vi "Arquivo de Configuração.vi"(0 "Caminho do arquivo":path, 1 "Modo":T2, 2 "Configurações":T1={"Simulações"={"Nível Qualidade"="avi", "Turno"="avi"}, "Captura de Imagens"={"Pasta com imagens"=path "", "Mostrar imagens capturadas"=FALSE}, "Caminhos"={"Arquivo de configuração"=path ""}}, 3 "error in (no error)":errorcluster) -> (9 "Configurações 2":T1={"Simulações"={"Nível Qualidade"="avi", "Turno"="avi"}, "Captura de Imagens"={"Pasta com imagens"=path "", "Mostrar imagens capturadas"=FALSE}, "Caminhos"={"Arquivo de configuração"=path ""}}, 10 "error out":errorcluster)   [LabVIEW 2020, in "Configurações.lvlib"]
uses:
  <vilib>/Utility/config.llb/Read Key (I32).vi
  <vilib>/Utility/config.llb/Write Key (I32).vi
  <vilib>/Utility/config.llb/Read Key (Path).vi
  <vilib>/Utility/config.llb/Write Key (Path).vi
  <vilib>/Utility/config.llb/Read Key (Boolean).vi
  <vilib>/Utility/config.llb/Write Key (Boolean).vi
  <vilib>/Utility/config.llb/Read Key (String).vi
  <vilib>/Utility/config.llb/Write Key (String).vi
  <vilib>/Utility/config.llb/NI_LVConfig.lvlib
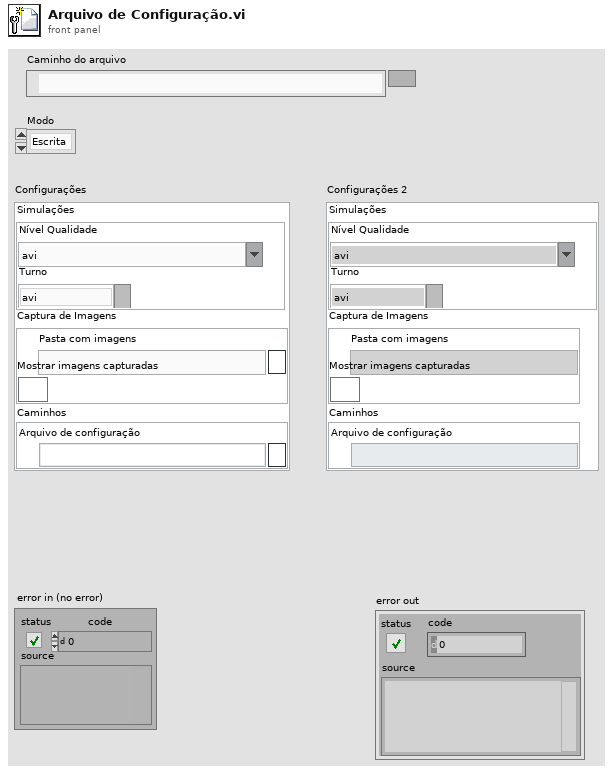
[diagram p1: front panel]
types:
  T1 = typedef "Configurações.lvlib/Configurações padrões.ctl" = cluster{"Simulações":cluster{"Nível Qualidade":string, "Turno":string}, "Captura de Imagens":cluster{"Pasta com imagens":path, "Mostrar imagens capturadas":bool}, "Caminhos":cluster{"Arquivo de configuração":path}}
  T2 = typedef "Ações de configuração 2.ctl" = enum16{"Escrita", "Leitura"}
  T3 = typedef "NI_LVConfig.lvlib/Config Data RefNum.ctl" = refnum<k1>
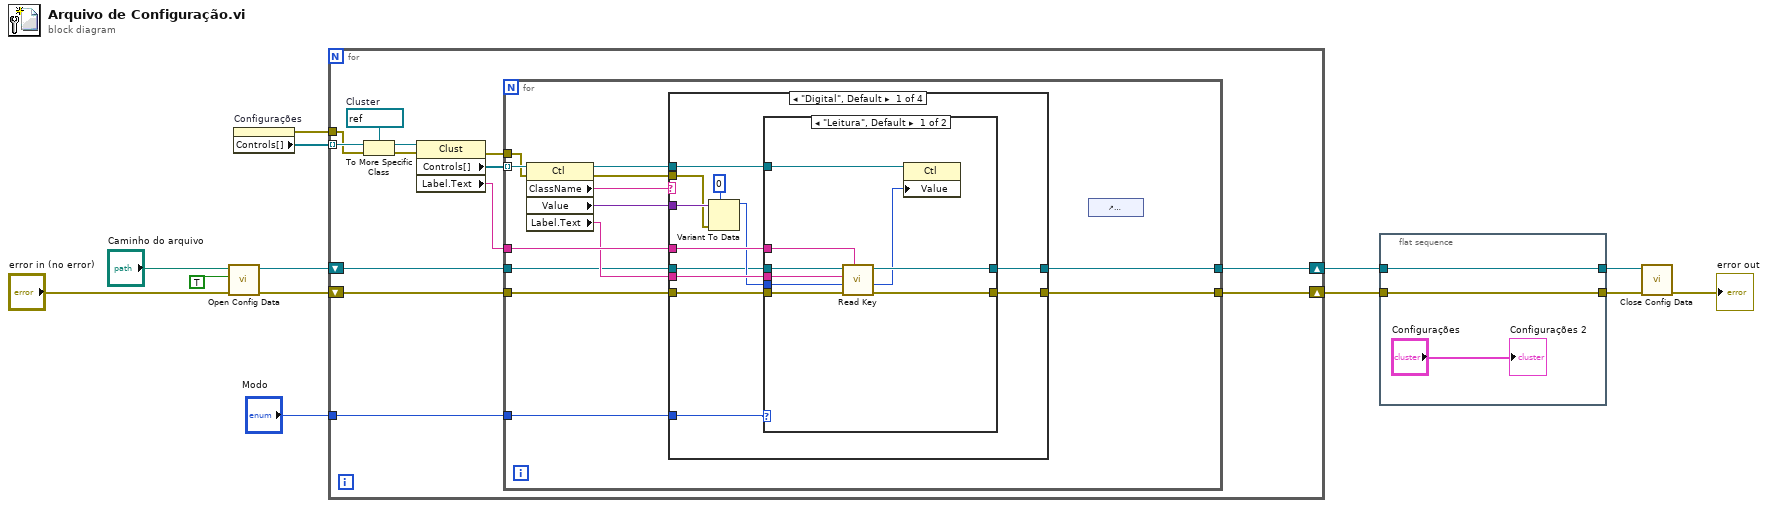
[diagram p0: block diagram]
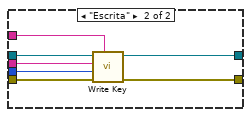
[diagram p2: hidden frame]
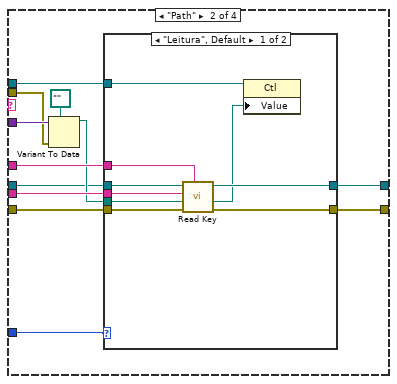
[diagram p3: hidden frame]
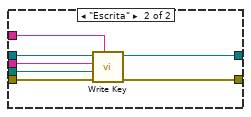
[diagram p4: hidden frame]
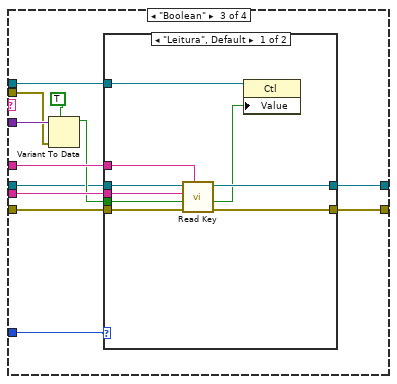
[diagram p5: hidden frame]
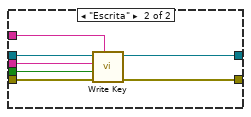
[diagram p6: hidden frame]
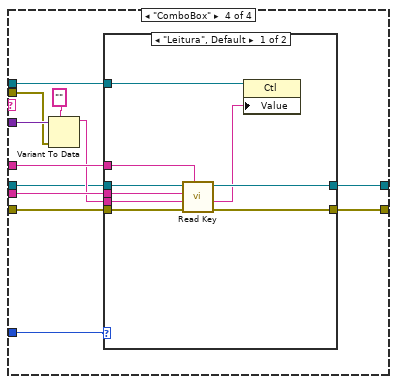
[diagram p7: hidden frame]
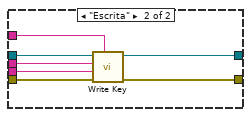
[diagram p8: hidden frame]
diagram:
  n1 = call <vilib>:"Open Config Data.vi"("error in (no error)"="error in (no error)", "create file if necessary (T)"=TRUE, "configuration file path"="Caminho do arquivo") -> ("error out"=w11:errorcluster, "refnum"=w12:T3)  [unwired: 6 in, 1 out]
  n2 = property on="Configurações" class="Clust (strict)"() -> (error out=w5:errorcluster, "Controls[]"=w9:refnum<vi>[])  [unwired: 2 in, 1 out]
  n3 = for {
    shift-right: [w18] -> w3
    shift-left: w12 -> [w19]
    shift-right: [w16] -> w1
    shift-left: w11 -> [w17]
    tunnel: w9 -> [w25] mode=indexing
    tunnel: "Modo" -> [w15]
    tunnel: w5 -> [w14]
    w26 = refnum<vi> refnum  # Cluster
    n4 = To More Specific Class(target class=w26, reference=w25, error in=w14) -> (specific class reference=w24:refnum<vi>, error out=w23:errorcluster)
    n5 = property class="Clust"(reference=w24, error in=w23) -> (error out=w21:errorcluster, "Controls[]"=w22:refnum<vi>[], "Label.Text"=w20:string)  [unwired: 1 out]
    n6 = for {
      tunnel: w22 -> [w39] mode=indexing
      tunnel: w21 -> [w36]
      tunnel: w20 -> [w34]
      tunnel: w19 -> [w32]
      tunnel: [w31] -> w18
      tunnel: w17 -> [w30]
      tunnel: [w29] -> w16
      tunnel: w15 -> [w28]
      n7 = property class="Ctl"(reference=w39, error in=w36) -> (reference out=w27:refnum<vi>, error out=w35:errorcluster, "ClassName"=w38:string, "Value"=w37:variant, "Label.Text"=w33:string)
      n8 = case shown="\"Digital\", Default" w38 {
        tunnel: w37 -> [w51 w79 w107 w135]
        tunnel: w35 -> [w50 w78 w106 w134]
        tunnel: w34 -> [w49 w77 w105 w133]
        tunnel: w33 -> [w48 w76 w104 w132]
        tunnel: w32 -> [w46 w74 w102 w130]
        tunnel: [w45 w73 w101 w129] -> w31
        tunnel: w30 -> [w44 w72 w100 w128]
        tunnel: [w43 w71 w99 w127] -> w29
        tunnel: w28 -> [w41 w70 w98 w126]
        tunnel: w27 -> [w40 w69 w97 w125]
        frame "Digital", Default {
          n9 = Variant To Data(error in=w50, type=0, Variant=w51) -> (data=w47:i32)  [unwired: 1 out]
          n10 = case shown="\"Leitura\", Default" w41 {
            tunnel: w49 -> [w53 w67]
            tunnel: w48 -> [w52 w66]
            tunnel: w47 -> [w56 w65]
            tunnel: w46 -> [w60 w64]
            tunnel: [w59 w63] -> w45
            tunnel: w44 -> [w58 w62]
            tunnel: [w57 w61] -> w43
            tunnel: w40 -> [w55 _]
            frame "Leitura", Default {
              n11 = call-poly <vilib>:"Read Key.vi"("section"=w53, "error in (no error)"=w58, "default value"=w56, "key"=w52, "refnum"=w60) -> ("error out"=w57:errorcluster, "value"=w54:i32, "refnum out"=w59:T3)  [unwired: 3 in, 1 out]
              n12 = property class="Ctl"(reference=w55, "Value"=w54) -> ()  [unwired: 1 in, 2 out]
            }
            frame "Escrita" {
              n13 = call-poly <vilib>:"Write Key.vi"("section"=w67, "error in (no error)"=w62, "value"=w65, "key"=w66, "refnum"=w64) -> ("error out"=w61:errorcluster, "refnum out"=w63:T3)  [unwired: 4 in, 1 out]
            }
          }
        }
        frame "Path" {
          n14 = Variant To Data(error in=w78, type=path "", Variant=w79) -> (data=w75:path)  [unwired: 1 out]
          n15 = case shown="\"Leitura\", Default" w70 {
            tunnel: w77 -> [w81 w95]
            tunnel: w76 -> [w80 w94]
            tunnel: w75 -> [w84 w93]
            tunnel: w74 -> [w88 w92]
            tunnel: [w87 w91] -> w73
            tunnel: w72 -> [w86 w90]
            tunnel: [w85 w89] -> w71
            tunnel: w69 -> [w83 _]
            frame "Leitura", Default {
              n16 = call-poly <vilib>:"Read Key.vi"("section"=w81, "error in (no error)"=w86, "default value"=w84, "key"=w80, "refnum"=w88) -> ("error out"=w85:errorcluster, "value"=w82:path, "refnum out"=w87:T3)  [unwired: 3 in, 1 out]
              n17 = property class="Ctl"(reference=w83, "Value"=w82) -> ()  [unwired: 1 in, 2 out]
            }
            frame "Escrita" {
              n18 = call-poly <vilib>:"Write Key.vi"("section"=w95, "error in (no error)"=w90, "value"=w93, "key"=w94, "refnum"=w92) -> ("error out"=w89:errorcluster, "refnum out"=w91:T3)  [unwired: 4 in, 1 out]
            }
          }
        }
        frame "Boolean" {
          n19 = Variant To Data(error in=w106, type=TRUE, Variant=w107) -> (data=w103:bool)  [unwired: 1 out]
          n20 = case shown="\"Leitura\", Default" w98 {
            tunnel: w105 -> [w109 w123]
            tunnel: w104 -> [w108 w122]
            tunnel: w103 -> [w112 w121]
            tunnel: w102 -> [w116 w120]
            tunnel: [w115 w119] -> w101
            tunnel: w100 -> [w114 w118]
            tunnel: [w113 w117] -> w99
            tunnel: w97 -> [w111 _]
            frame "Leitura", Default {
              n21 = call-poly <vilib>:"Read Key.vi"("section"=w109, "error in (no error)"=w114, "default value"=w112, "key"=w108, "refnum"=w116) -> ("error out"=w113:errorcluster, "value"=w110:bool, "refnum out"=w115:T3)  [unwired: 3 in, 1 out]
              n22 = property class="Ctl"(reference=w111, "Value"=w110) -> ()  [unwired: 1 in, 2 out]
            }
            frame "Escrita" {
              n23 = call-poly <vilib>:"Write Key.vi"("section"=w123, "error in (no error)"=w118, "value"=w121, "key"=w122, "refnum"=w120) -> ("error out"=w117:errorcluster, "refnum out"=w119:T3)  [unwired: 4 in, 1 out]
            }
          }
        }
        frame "ComboBox" {
          n24 = Variant To Data(error in=w134, type="", Variant=w135) -> (data=w131:string)  [unwired: 1 out]
          n25 = case shown="\"Leitura\", Default" w126 {
            tunnel: w133 -> [w137 w151]
            tunnel: w132 -> [w136 w150]
            tunnel: w131 -> [w140 w149]
            tunnel: w130 -> [w144 w148]
            tunnel: [w143 w147] -> w129
            tunnel: w128 -> [w142 w146]
            tunnel: [w141 w145] -> w127
            tunnel: w125 -> [w139 _]
            frame "Leitura", Default {
              n26 = call-poly <vilib>:"Read Key.vi"("section"=w137, "error in (no error)"=w142, "default value"=w140, "key"=w136, "refnum"=w144) -> ("error out"=w141:errorcluster, "value"=w138:string, "refnum out"=w143:T3)  [unwired: 3 in, 1 out]
              n27 = property class="Ctl"(reference=w139, "Value"=w138) -> ()  [unwired: 1 in, 2 out]
            }
            frame "Escrita" {
              n28 = call-poly <vilib>:"Write Key.vi"("section"=w151, "error in (no error)"=w146, "value"=w149, "key"=w150, "refnum"=w148) -> ("error out"=w145:errorcluster, "refnum out"=w147:T3)  [unwired: 4 in, 1 out]
            }
          }
        }
      }
      n29 = control-ref of="Configurações"() -> ()  [unwired: 1 out]
    }
  }
  n30 = flat-sequence {
    tunnel: [w153] -> w4
    tunnel: w3 -> [w153]
    tunnel: [w152] -> w2
    tunnel: w1 -> [w152]
    frame #0 {
      "Configurações 2" <- "Configurações"
    }
  }
  n31 = call <vilib>:"Close Config Data.vi"("error in (no error)"=w2, "refnum"=w4) -> ("error out"=→"error out":errorcluster)  [unwired: 8 in, 1 out]
